vi "Write Formatted Data.vi"(8 "error in (no error)":errorcluster, 10 "Formatted Data":string, 11 "Stream in":refnum<class "Stream.lvclass">) -> (0 "error out":errorcluster, 3 "Stream out":refnum<class "Stream.lvclass">)   [LabVIEW 2020, in "Stream.lvlib" / "Stream.lvclass"]
uses:
  Stream.lvclass
  Data Direction.ctl
  Stream.lvlib
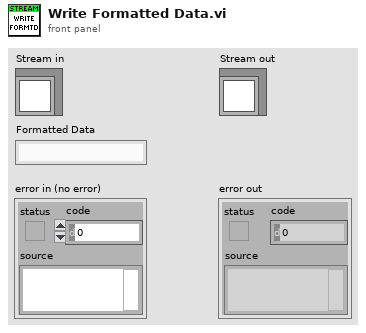
[diagram p1: front panel]
types:
  T1 = typedef "Stream.lvlib/Data Direction.ctl" = enum16{"Incoming", "Outgoing"}
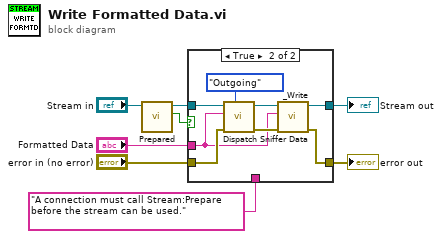
[diagram p0: block diagram]
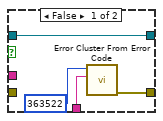
[diagram p2: hidden frame]
diagram:
  n1 = call "Prepared.vi"("Stream in"="Stream in") -> ("Prepared"=w5:bool, "Stream out"=w4:refnum<class "Stream.lvclass">)  [unwired: 8 in, 1 out]
  n2 = case shown="True" w5 {
    tunnel: [w12 w18] -> w2
    tunnel: w4 -> [w12 w17]
    tunnel: "A connection must call Stream:Prepare before the stream can be used." ("error message (\"\")") -> [w10 _]
    tunnel: "error in (no error)" -> [_ w15]
    tunnel: "Formatted Data" -> [_ w13]
    tunnel: [w9 w14] -> w7
    frame False {
      n3 = call <vilib>:"Error Cluster From Error Code.vi"("error message (\"\")"=w10, "error code (0)"=363522) -> ("error out"=w9:errorcluster)  [unwired: 7 in]
    }
    frame True {
      n4 = call "Dispatch Sniffer Data.vi"("Data Direction"=Data_Direction."Outgoing", "error in (no error)"=w15, "Data"=w13, "Stream in"=w17) -> ("error out"=w16:errorcluster, "Stream out"=w19:refnum<class "Stream.lvclass">)  [unwired: 6 in]
      n5 = call-dynamic "_Write.vi"("error in (no error)"=w16, "Data"=w13, "Stream in"=w19) -> ("error out"=w14:errorcluster, "Stream out"=w18:refnum<class "Stream.lvclass">)  [unwired: 7 in]
    }
  }
  "error out" <- w7
  "Stream out" <- w2
